vi "Word_Set_Orientation.vi"(0 "Word._Document":refnum<k7>, 7 "orientation (portrait)":u16, 11 "error in":errorcluster) -> (15 "error out":errorcluster)   [LabVIEW 2010, in "NI_ReportGenerationToolkit.lvlib"]
uses:
  <vilib>/addons/_office/NI_ReportGenerationToolkit.lvlib
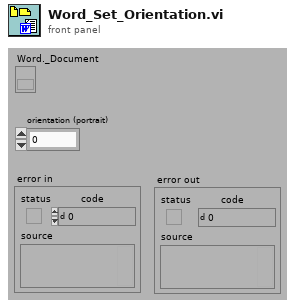
[diagram p1: front panel]
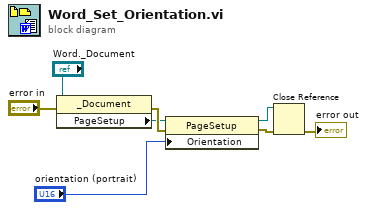
[diagram p0: block diagram]
diagram:
  n1 = property class="_Document"(reference="Word._Document", error in="error in") -> (error out=w6:errorcluster, "PageSetup"=w1:refnum<k7>)  [unwired: 1 out]
  n2 = property class="PageSetup"(reference=w1, error in=w6, "Orientation"="orientation (portrait)") -> (reference out=w3:refnum<k7>, error out=w2:errorcluster)
  n3 = Close Reference(reference=w3, error in (no error)=w2) -> (error out=→"error out":errorcluster)
